vi "Load Calibration from User Input.vi"(7 "path":string, 8 "error in (no error)":errorcluster, 10 "Old values":T1, 11 "PathControl in":refnum<class "PathControl.lvclass">) -> (0 "error out":errorcluster, 3 "PathControl out":refnum<class "PathControl.lvclass">)   [LabVIEW 2020, in "PathControl.lvclass"]
uses:
  PathControl.lvclass
  Measurements Specific Paths.ctl
  Paths.ctl
panel:
  in  "Empty Data Table":bool
  out "Path":T2
  out "Measurement specfic paths":T3=enum."Harmonics"
  in  "Cancel Button":bool
  in  "OK Button":bool
  in  "FreqLoss":dbl[][](array[numeric]) caption="Frequency (MHz) | Gain (dB)"
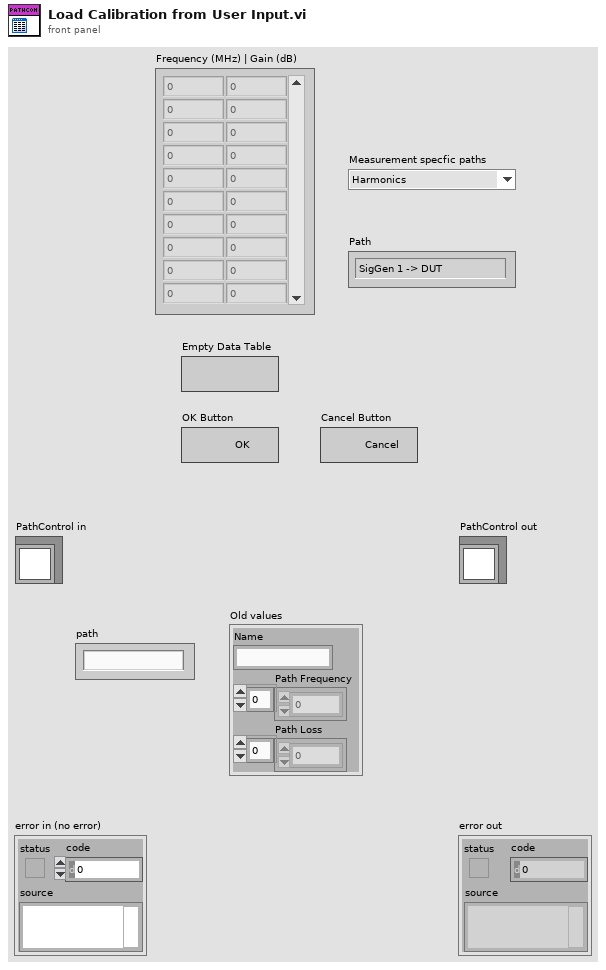
[diagram p1: front panel]
types:
  T1 = cluster{"Name":string, "Path Frequency":dbl[], "Path Loss":dbl[]}
  T2 = typedef "PathControl.lvclass/Paths.ctl" = enum16{"SigGen 1 -> DUT", "SigGen 2 -> DUT", "SigGen 1 -> PM 1", "SigGen 1 -> PM 2", "DUT -> SA", "DUT -> PM 2", "VSG -> DUT", "SigGen 2 -> PM 1", "SigGen 2 -> PM 2"}
  T3 = typedef "PathControl.lvclass/Measurements Specific Paths.ctl" = enum16{"No calibration", "Harmonics", "IMD", "S Parameter", "AM-AM", "MCCW-ACLR", "DC", "LCR", "Power Meter GUI", "RF Power"}
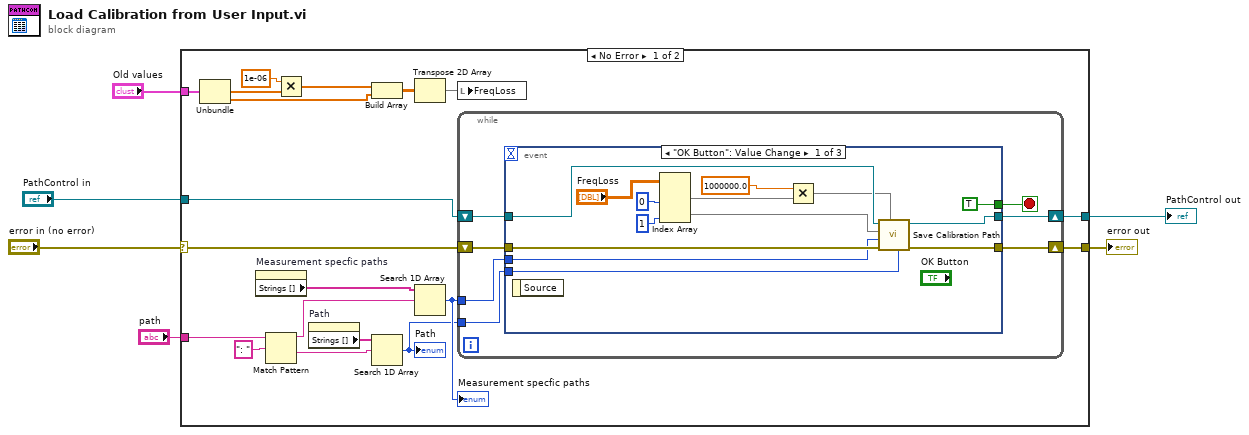
[diagram p0: block diagram]
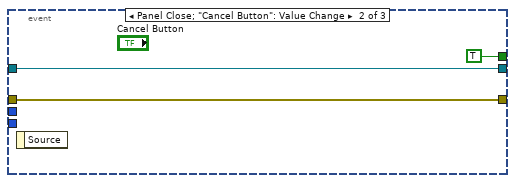
[diagram p2: hidden frame]
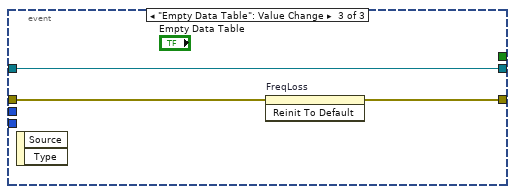
[diagram p3: hidden frame]
diagram:
  n1 = case shown="No Error" "error in (no error)" {
    selector: "error in (no error)" -> [w23 w54]
    tunnel: [w22 w54] -> w5
    tunnel: [w24 w53] -> w3
    tunnel: "PathControl in" -> [w25 w53]
    tunnel: "Old values" -> [w21 _]
    tunnel: "path" -> [w13 _]
    frame No Error {
      n2 = Unbundle(w21) -> ("Path Frequency"=w16:dbl[], "Path Loss"=w20:dbl[])  [unwired: 1 out]
      n3 = property on="Measurement specfic paths" class="Enum (strict)"() -> ("Strings []"=w10:string[])  [unwired: 2 in, 2 out]
      n4 = Match Pattern(string=w13, regular expression=": ") -> (before substring=w12:string, after substring=w11:string)  [unwired: 1 in, 2 out]
      n5 = Multiply(x=1e-06, y=w16) -> (x*y=w15:dbl[])
      n6 = property on="Path" class="Enum (strict)"() -> ("Strings []"=w9:string[])  [unwired: 2 in, 2 out]
      n7 = Build Array(w15, w20) -> (w19:dbl[][])
      n8 = Search 1D Array(1D array=w9, element=w11) -> (index of element=w7:i32)  [unwired: 1 in]
      "Path" <- w7
      n9 = Transpose 2D Array(2D array=w19) -> (transposed array=w18:dbl[][])
      n10 = Search 1D Array(1D array=w10, element=w12) -> (index of element=w8:i32)  [unwired: 1 in]
      "Measurement specfic paths" <- w8
      n11 = local write "FreqLoss"(w18) -> ()
      n12 = while {
        shift-right: [w30] -> w24
        shift-left: w25 -> [w31]
        shift-right: [w28] -> w22
        shift-left: w23 -> [w29]
        tunnel: w8 -> [w27]
        tunnel: w7 -> [w26]
        stop <- w32 stop-if-true
        n13 = event shown="[0] \"OK Button\": Value Change" {
          selector: _ -> [_ _ _]
          dyn-events: _ -> [_ _ _]
          timeout: _ -> [_ _ _]
          tunnel: [TRUE TRUE _] -> w32
          tunnel: w31 -> [w45 w47 w51]
          tunnel: [w44 w47 w51] -> w30
          tunnel: w29 -> [w43 w48 w52]
          tunnel: [w42 w48 w50] -> w28
          tunnel: w27 -> [w34 _ _]
          tunnel: w26 -> [w33 _ _]
          event "OK Button": Value Change {
            n14 = event-data() -> ()  [unwired: 1 in, 1 out]
            n15 = Index Array(array="FreqLoss", index (col) #1=0 ("disabled index (col)"), index (col) #2=1 ("index (col)")) -> (element #1=w39:dbl[], element #2=w40:dbl[])  [unwired: 2 in]
            n16 = Multiply(x=1000000.0, y=w39) -> (x*y=w38:dbl[])
            n17 = call "Save Calibration Path.vi"("Path"=w33, "Frequency"=w38, "Error In"=w43, "Measurement specfic paths"=w34, "Path Loss"=w40, "PathControl in"=w45) -> ("Error Out"=w42:errorcluster, "PathControl out"=w44:refnum<class "PathControl.lvclass">)  [unwired: 4 in]
          }
          event Panel Close; "Cancel Button": Value Change {
            n18 = event-data() -> ()  [unwired: 1 in, 1 out]
          }
          event "Empty Data Table": Value Change {
            n19 = event-data() -> ()  [unwired: 1 in, 2 out]
            n20 = invoke on="FreqLoss" class="Arr (strict)" method="Reinit To Default"(error in=w52) -> (error out=w50:errorcluster)  [unwired: 2 in, 2 out]
          }
        }
      }
    }
    frame Error {
    }
  }
  "error out" <- w5
  "PathControl out" <- w3
